vi "Example TX.vi"(0 "Network API":refnum<class "niInstr Network API FPGA v1.lvclass">, 1 "FIFO In":refnum<k21>, 5 "Controls":T3={"UDP Source Port"=43981, "UDP Destination Port"=61185, "preferred datagram size"=1400, "Use Pattern Gen"=FALSE, "max frame payload"=1472, "minimum packet interval"=1, "stream.num samples 0"=0, "stream.request state 0"=enum."Idle"} {"UDP Destination Port" format="%04x"; "UDP Source Port" format="%04x"}) -> (6 "Indicators":T1)   [LabVIEW 2017, in "My Network FPGA v1.lvlib"]
uses:
  My Network FPGA v1.lvlib
  <instrlib>/_niInstr/Network/API/v1/FPGA/niInstr Network API FPGA v1.lvclass
  TX Controls.ctl
  <instrlib>/_niInstr/Streaming/v1/Common/Stream State.ctl
  TX Indicators.ctl
  <vilib>/rvi/DataTransferAndStorage/Container/Common/niFpgaContainerExecOnDevCompGetState.vi
  <vilib>/rvi/Emulation/niFpgaSctlEmulationGetInTimedLoop.vi
  <vilib>/rvi/errors/niFpgaSetErrorForExecOnDevCompSimple.vi
  <vilib>/rvi/eio/common/nirviEmuReportErrorAndStop.vi
  <vilib>/rvi/interface/RandomDataEmulation/nirviRandomDataAcquireLock.vi
  <vilib>/rvi/interface/RandomDataEmulation/nirviRandomDataQueueStore.vi
  <vilib>/rvi/interface/RandomDataEmulation/nirviRandomDataReleaseLock.vi
  <vilib>/rvi/interface/RandomDataEmulation/nirviFPGAContextMergeError.vi
  <vilib>/rvi/interface/RandomDataEmulation/nirviRandomDataCheckExitLoopConditions.vi
  <vilib>/express/rvi/timingcommon/nirviCommon.vi
  <vilib>/rvi/interface/RandomDataEmulation/niFpgaRandomDataHandleErrors.vi
  <vilib>/rvi/DataTransferAndStorage/Container/XNode/niFpgaContainer.xnode
  <vilib>/rvi/FIFO/Fifo_Resource/niFpgaFifoEmulationRefInMultiElement.vi
  <instrlib>/_niInstr/Network/Ethernet/Utility/v1/FPGA/niInstr Ethernet Utilities FPGA v1.lvlib
  <instrlib>/_niInstr/Streaming/v1/FPGA/niInstr Streaming v1 FPGA.lvlib
  <instrlib>/_niInstr/Streaming/v1/Common/niInstr Streaming v1 Common.lvlib
  <instrlib>/_niInstr/Network/Ethernet/MAC/Raw Stream/v1/niInstr Ethernet MAC Raw Stream v1.lvclass
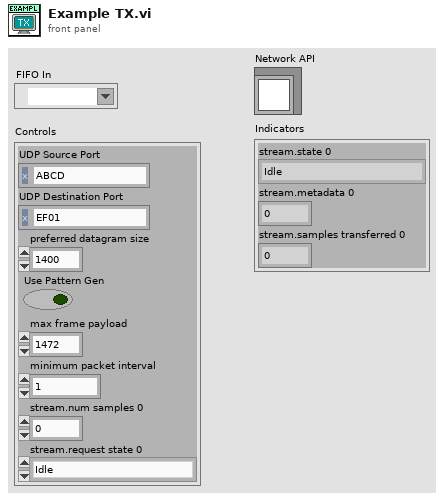
[diagram p1: front panel]
types:
  T1 = typedef "My Network FPGA v1.lvlib/TX Indicators.ctl" = cluster{"stream.state 0":T2, "stream.metadata 0":u64, "stream.samples transferred 0":u64}
  T2 = typedef "niInstr Streaming v1 Common.lvlib/Stream State.ctl" = enum8{"Idle", "Finite Transfer", "Continuous", "Done", "Error", "Not Ready", "Cancel"}
  T3 = typedef "My Network FPGA v1.lvlib/TX Controls.ctl" = cluster{"UDP Source Port":u16, "UDP Destination Port":u16, "preferred datagram size":u16, "Use Pattern Gen":bool, "max frame payload":u16, "minimum packet interval":u32, "stream.num samples 0":u64, "stream.request state 0":T2}
  T4 = cluster{"ready for input (payload data)":bool, "ready for input (start packet)":bool}
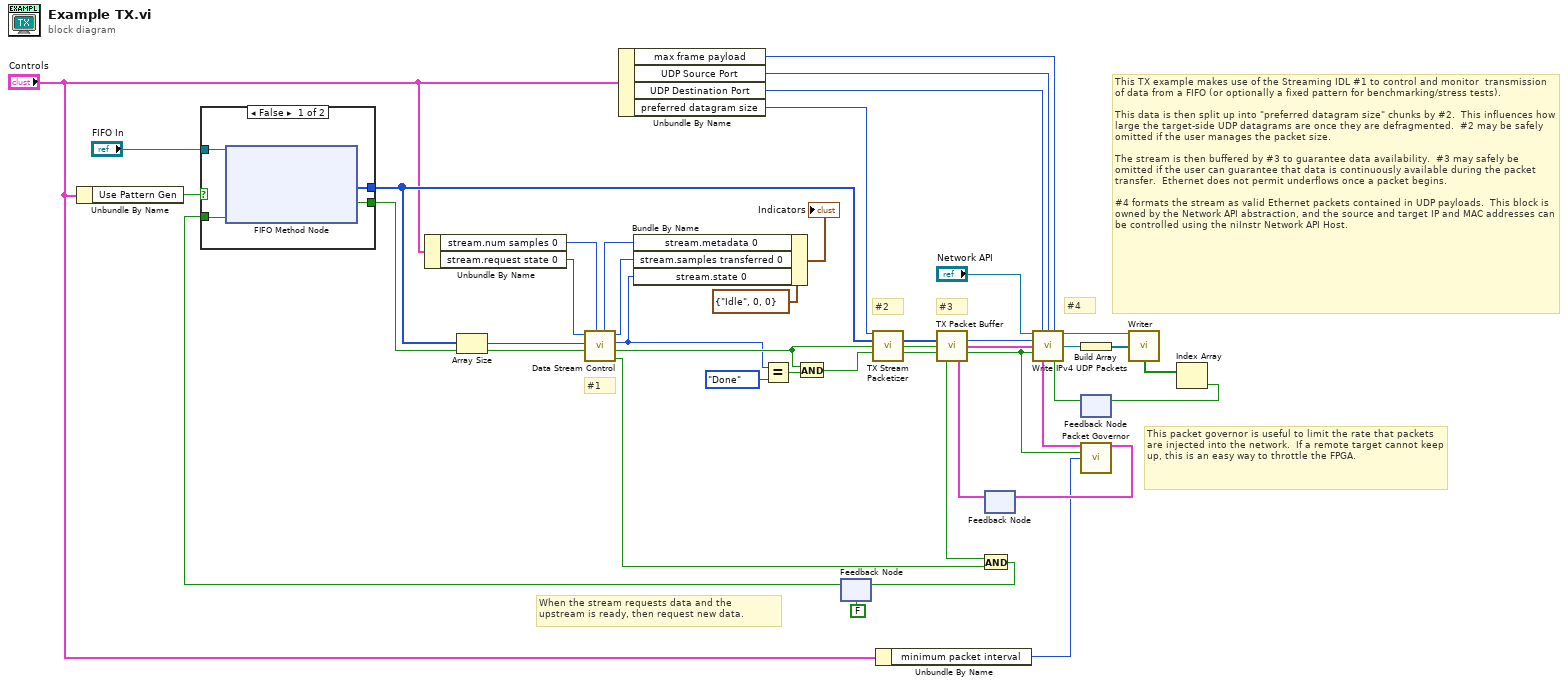
[diagram p0: block diagram]
diagram:
  # "#4"
  # "#3"
  # "#2"
  # "When the stream requests data and the upstream is ready, then request new data."
  # "#1"
  # "This TX example makes use of the Streaming IDL #1 to control and monitor  transmission of data from a FIFO (or optionally a fixed pattern for benchmarking/stress tests).\n\nThis data is then split up into \"preferred datagram size\" chunks by #2.  This influences how large the target-side UDP datagrams are once they are defragmented.  #2 may be safely omitted if the user manages the packet size.\n\nThe stream is then buffered by #3 to guarantee data availability.  #3 may safely be omitted if the user can guarantee that data is continuously available during the packet transfer.  Ethernet does not permit underflows once a packet begins.\n\n#4 formats the stream as valid Ethernet packets contained in UDP payloads.  This block is owned by the Network API abstraction, and the source and target IP and MAC addresses can be controlled using the niInstr Network API Host."
  # "This packet governor is useful to limit the rate that packets are injected into the network.  If a remote target cannot keep up, this is an easy way to throttle the FPGA."
  n1 = Unbundle By Name("Controls") -> ("Use Pattern Gen"=w9:bool)
  n2 = Unbundle By Name("Controls") -> ("stream.num samples 0"=w8:u64, "stream.request state 0"=w7:T2)
  n3 = Unbundle By Name("Controls") -> ("max frame payload"=w5:u16, "UDP Source Port"=w4:u16, "UDP Destination Port"=w3:u16, "preferred datagram size"=w6:u16)
  n4 = feedback #1(FALSE ("ready for input")) -> (w35:bool)
  n5 = case shown="False" w9 {
    tunnel: "FIFO In" -> [w47 _]
    tunnel: [w46 _] -> w22
    tunnel: w35 -> [w45 w48]
    tunnel: [w44 w48] -> w34
    frame False {
      n6 = xnode ("FIFO Method Node")("Ready for Output"=w45, "FIFO In"=w47) -> ("Element"=w46:u8[], "Output Valid"=w44:bool)  [unwired: 1 out]
    }
    frame True {
    }
  }
  n7 = Array Size(array=w22) -> (size(s)=w21:i32)
  n8 = call <instrlib>:"Data Stream Control.vi"("stream.num samples 0"=w8, "data valid"=w34, "element count"=w21, "stream.request state 0"=w7) -> ("request data"=w16:bool, "send data"=w31:bool, "stream.state 0"=w10:T2, "stream.samples transferred 0"=w11:u64, "stream.metadata 0"=w12:u64)  [unwired: 3 in]
  n9 = Bundle By Name(cluster=T1 {"stream.state 0"=enum."Idle", "stream.metadata 0"=0, "stream.samples transferred 0"=0} ("Indicators"), "stream.metadata 0"=w12, "stream.samples transferred 0"=w11, "stream.state 0"=w10) -> (→"Indicators":T1)
  n10 = Equal?(x=w10, y=Stream_State."Done" ("stream.state 0")) -> (x = y?=w32:bool)
  n11 = And(x=w31, y=w32) -> (x .and. y?=w30:bool)
  n12 = call <instrlib>:"TX Stream Packetizer.vi"("preferred datagram size"=w6, "data in"=w22, "data valid in"=w31, "last in"=w30) -> ("data out"=w38:u8[], "data valid out"=w40:bool, "last out"=w39:bool)  [unwired: 8 in, 1 out]
  n13 = Unbundle By Name("Controls") -> ("minimum packet interval"=w1:u32)
  n14 = feedback #2() -> (w36:T4)  [unwired: 1 in]
  n15 = call <instrlib>:"TX Packet Buffer.vi"("data"=w38, "data valid"=w40, "last/flush"=w39, "ready for output?"=w36) -> ("tx bytes to send"=w29:u16, "output data"=w37:cluster{"data":u8[], "data valid":bool}, "start packet"=w18:bool, "ready for input"=w17:bool)  [unwired: 8 in]
  n16 = And(x=w17, y=w16) -> (x .and. y?=w15:bool)
  n17 = feedback-in #1(w15) -> ()
  n18 = feedback #3() -> (w26:bool)  [unwired: 1 in]
  n19 = call <instrlib>:"Write IPv4 UDP Packets.vi"("niInstr Network API FPGA v1.lvclass"="Network API", "UDP destination port"=w3, "UDP source port"=w4, "max frame payload"=w5, "total datagram payload"=w29, "data"=w37, "start packet"=w18, "ready for output"=w26) -> ("niInstr Network API FPGA v1.lvclass out"=w24:refnum<class "niInstr Network API FPGA v1.lvclass">, "niInstr Ethernet MAC Raw Stream v1 out"=w25:refnum<class "niInstr Ethernet MAC Raw Stream v1.lvclass">, "ready for input?"=w19:T4)  [unwired: 5 in]
  n20 = Build Array(w25) -> (w28:refnum<class "niInstr Ethernet MAC Raw Stream v1.lvclass">[])
  n21 = call "Packet Governor.vi"("ready for input? in"=w19, "start packet"=w18, "minimum packet interval"=w1) -> ("ready for input? out"=w20:T4)  [unwired: 12 in]
  n22 = feedback-in #2(w20) -> ()
  n23 = call <instrlib>:"Writer.vi"("niInstr Network API FPGA v1.lvclass"=w24, "input packet streams"=w28) -> ("ready for input"=w27:bool[])  [unwired: 13 in]
  n24 = Index Array(array=w27) -> (element=w41:bool)  [unwired: 1 in]
  n25 = feedback-in #3(w41) -> ()
